vi "报警XML解析.vi"(8 "error in (no error)":errorcluster caption="错误输入（无错误）", 11 "筛选输入":T1={"componentParent"="斯坦道营养盐", "equipVersion"="B", "Code"=""}) -> (0 "error out":errorcluster caption="错误输出", 3 "data":T2(array[cluster]))   [LabVIEW 2016, in "Alarm interface.lvlib"]
uses:
  Alarm interface.lvlib
  <vilib>/xml/Load XML File.vi
  <vilib>/xml/Close Reference(Node).vi
  <vilib>/xml/NI_XML.lvlib
  <resource>/objmgr/DOMUserDefRef.rc
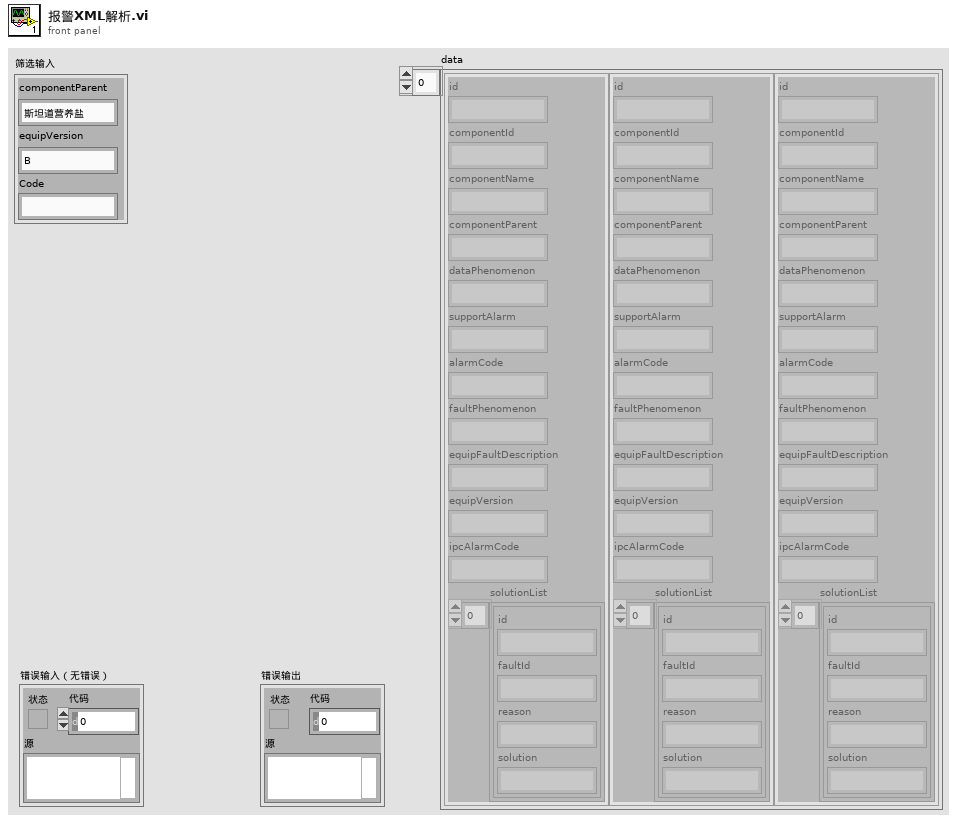
[diagram p1: front panel]
types:
  T1 = cluster{"componentParent":string, "equipVersion":string, "Code":string}
  T2 = cluster{"id":string, "componentId":string, "componentName":string, "componentParent":string, "dataPhenomenon":string, "supportAlarm":string, "alarmCode":string, "faultPhenomenon":string, "equipFaultDescription":string, "equipVersion":string, "ipcAlarmCode":string, "solutionList":cluster{"id":string, "faultId":string, "reason":string, "solution":string}[]}[]
  T3 = cluster{"node text":string, "node text":string, "node text":string, "node text":string}
  T4 = cluster{"id":string, "componentId":string, "componentName":string, "componentParent":string, "dataPhenomenon":string, "supportAlarm":string, "alarmCode":string, "faultPhenomenon":string, "equipFaultDescription":string, "equipVersion":string, "ipcAlarmCode":string, "solutionList":cluster{"id":string, "faultId":string, "reason":string, "solution":string}[]}
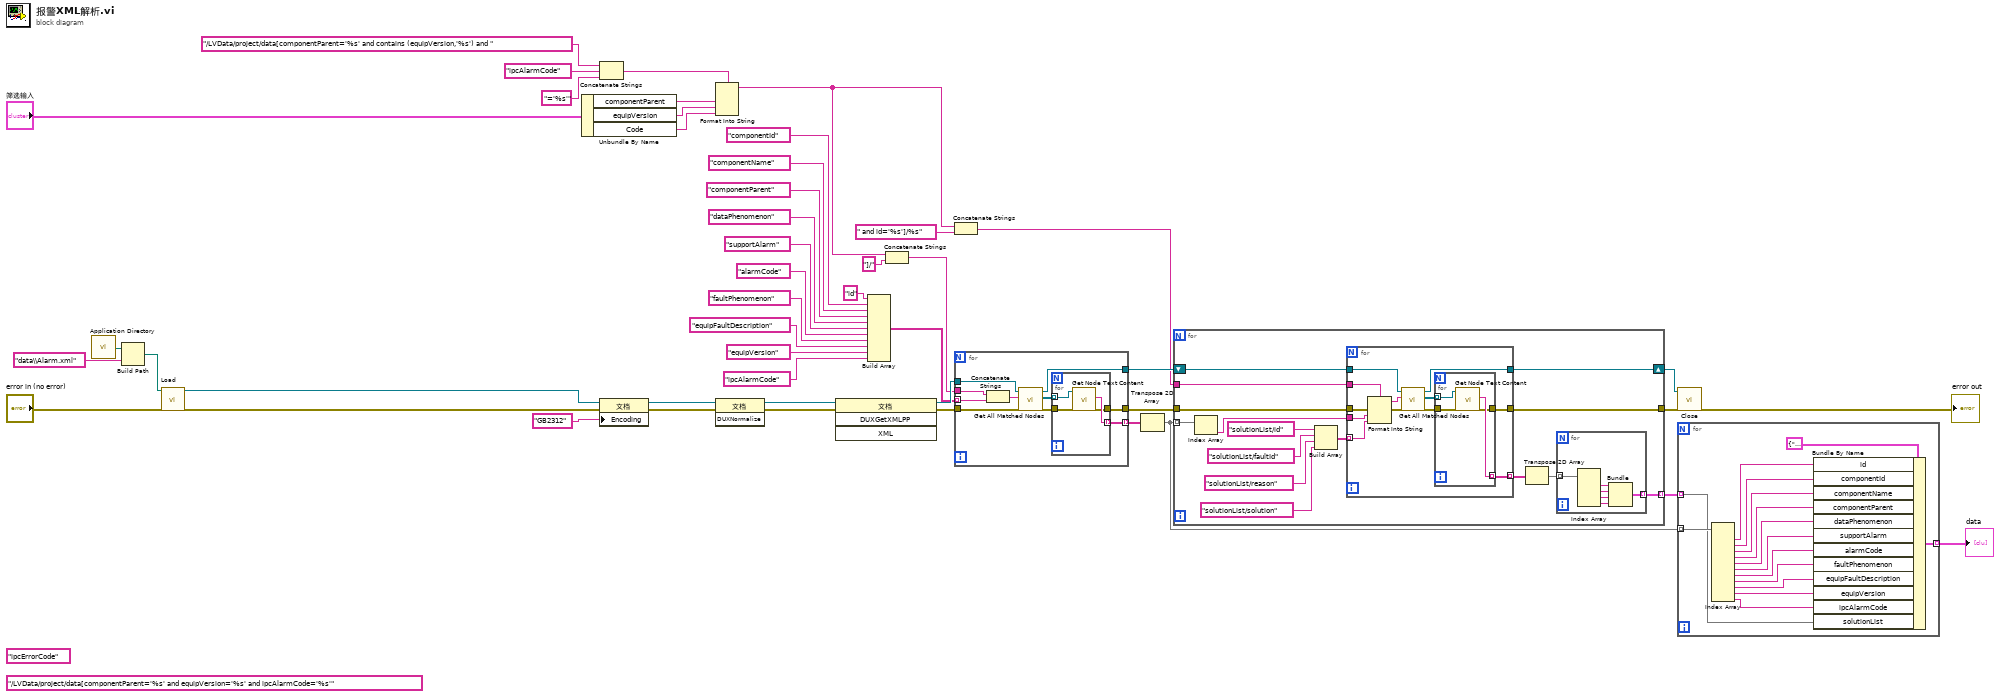
[diagram p0: block diagram]
diagram:
  (unwired) "/LVData/project/data[componentParent='%s' and equipVersion='%s' and ipcAlarmCode='%s'" ("格式字符串")
  (unwired) "ipcErrorCode"
  n1 = call <vilib>:"Application Directory.vi"() -> ("Application Directory"=w6:path)
  n2 = Build Path(base path=w6, name or relative path="data\\Alarm.xml" ("字符串")) -> (appended path=w4:path)
  n3 = call-poly <vilib>:"Load.vi"("path to XML document"=w4, "error in (no error)"="error in (no error)") -> ("DOM document out"=w44:refnum<k20>, "error out"=w43:errorcluster)  [unwired: 11 in, 1 out]
  n4 = Unbundle By Name("筛选输入") -> ("componentParent"=w10:string, "equipVersion"=w9:string, "Code"=w7:string)
  n5 = Concatenate Strings("/LVData/project/data[componentParent='%s' and contains (equipVersion,'%s') and " ("字符串"), "ipcAlarmCode", "='%s'" ("字符串")) -> (w8:string)
  n6 = property on="属性节点" class="文档"(reference=w44, error in=w43, "Encoding"="GB2312" ("文档编码")) -> (reference out=w46:refnum<k20>, error out=w45:errorcluster)
  n7 = Format Into String(format string=w8, w10, w9, w7) -> (resulting string=w2:string)  [unwired: 2 in, 1 out]
  n8 = invoke on="调用节点" class="文档" method="DUXNormalize"(reference=w46, error in=w45) -> (reference out=w42:refnum<k20>, error out=w41:errorcluster)  [unwired: 1 in, 1 out]
  n9 = invoke on="调用节点" class="文档" method="DUXGetXMLPP"(reference=w42, error in=w41) -> (reference out=w30:refnum<k20>, error out=w16:errorcluster)  [unwired: 2 in, 2 out]
  n10 = Build Array("id", "componentId", "componentName", "componentParent", "dataPhenomenon", "supportAlarm", "alarmCode", "faultPhenomenon", "equipFaultDescription", "equipVersion", "ipcAlarmCode") -> (w29:string[])
  n11 = Concatenate Strings(w2, "]/" ("字符串")) -> (w21:string)
  n12 = Concatenate Strings(w2, " and id='%s']/%s" ("字符串")) -> (w19:string)
  n13 = for {
    tunnel: w30 -> [w57]
    tunnel: w21 -> [w51]
    tunnel: w29 -> [w50] mode=indexing
    tunnel: [w55] -> w28 mode=indexing
    tunnel: [w54] -> w27
    tunnel: [w52] -> w17
    tunnel: w16 -> [w49]
    n14 = Concatenate Strings(w51, w50) -> (w48:string)
    n15 = call <vilib>:"Get All Matched Nodes.vi"("error in (no error)"=w49, "XPath expression"=w48, "node in"=w57) -> ("error out"=w53:errorcluster, "node result array"=w56:refnum<k20>[], "node out"=w54:refnum<k20>)  [unwired: 6 in]
    n16 = for {
      tunnel: w56 -> [w61] mode=indexing
      tunnel: [w60] -> w55 mode=indexing
      tunnel: w53 -> [w59]
      tunnel: [w58] -> w52
      n17 = call <vilib>:"Get Node Text Content.vi"("error in (no error)"=w59, "node in"=w61) -> ("error out"=w58:errorcluster, "node text"=w60:string)  [unwired: 7 in, 1 out]
    }
  }
  n18 = Transpose 2D Array(2D array=w28) -> (transposed array=w24:string[][])
  n19 = for {
    tunnel: w24 -> [w76] mode=indexing
    tunnel: w19 -> [w75]
    tunnel: [w64] -> w25 mode=indexing
    tunnel: w17 -> [w63]
    tunnel: [w62] -> w15
    shift-right: [w66] -> w26
    shift-left: w27 -> [w73]
    n20 = Index Array(array=w76) -> (element=w74:string)  [unwired: 1 in]
    n21 = Build Array("solutionList/id" ("XPath expression"), "solutionList/faultId" ("XPath expression"), "solutionList/reason" ("XPath expression"), "solutionList/solution" ("XPath expression")) -> (w68:string[])
    n22 = for {
      tunnel: w75 -> [w94]
      tunnel: w74 -> [w93]
      tunnel: w68 -> [w92] mode=indexing
      tunnel: w73 -> [w90]
      tunnel: [w88] -> w67 mode=indexing
      tunnel: [w87] -> w66
      tunnel: w63 -> [w86]
      tunnel: [w83] -> w62
      n23 = Format Into String(format string=w94, error in=w86, w93, w92) -> (resulting string=w89:string, error out=w85:errorcluster)  [unwired: 1 in]
      n24 = call <vilib>:"Get All Matched Nodes.vi"("error in (no error)"=w85, "XPath expression"=w89, "node in"=w90) -> ("error out"=w84:errorcluster, "node result array"=w91:refnum<k20>[], "node out"=w87:refnum<k20>)  [unwired: 6 in]
      n25 = for {
        tunnel: w91 -> [w98] mode=indexing
        tunnel: [w97] -> w88 mode=indexing
        tunnel: w84 -> [w96]
        tunnel: [w95] -> w83
        n26 = call <vilib>:"Get Node Text Content.vi"("error in (no error)"=w96, "node in"=w98) -> ("error out"=w95:errorcluster, "node text"=w97:string)  [unwired: 7 in, 1 out]
      }
    }
    n27 = Transpose 2D Array(2D array=w67) -> (transposed array=w65:string[][])
    n28 = for {
      tunnel: w65 -> [w82] mode=indexing
      tunnel: [w77] -> w64 mode=indexing
      n29 = Index Array(array=w82) -> (element #1=w81:string, element #2=w80:string, element #3=w79:string, element #4=w78:string)  [unwired: 4 in]
      n30 = Bundle("node text"=w81, "node text"=w80, "node text"=w79, "node text"=w78) -> (w77:T3)  [unwired: 1 in]
    }
  }
  n31 = call-poly <vilib>:"Close.vi"("error in (no error)"=w15, "node"=w26) -> ("error out"=→"error out":errorcluster)  [unwired: 7 out]
  n32 = for {
    tunnel: w24 -> [w101] mode=indexing
    tunnel: [w102] -> w23 mode=indexing
    tunnel: w25 -> [w100] mode=indexing
    n33 = Index Array(array=w101) -> (element #1=w112:string, element #2=w111:string, element #3=w110:string, element #4=w109:string, element #5=w108:string, element #6=w107:string, element #7=w106:string, element #8=w105:string, element #9=w104:string, element #10=w103:string, element #11=w99:string)  [unwired: 11 in]
    n34 = Bundle By Name(cluster=T4 {"id"="", "componentId"="", "componentName"="", "componentParent"="", "dataPhenomenon"="", "supportAlarm"="", "alarmCode"="", "faultPhenomenon"="", "equipFaultDescription"="", "equipVersion"="", "ipcAlarmCode"="", "solutionList"=[]} ("data"), "id"=w112, "componentId"=w111, "componentName"=w110, "componentParent"=w109, "dataPhenomenon"=w108, "supportAlarm"=w107, "alarmCode"=w106, "faultPhenomenon"=w105, "equipFaultDescription"=w104, "equipVersion"=w103, "ipcAlarmCode"=w99, "solutionList"=w100) -> (w102:T4)
  }
  "data" <- w23
